vi "GEA2 Commands Dishwasher Send Receive.vi"(7 "Input Data":T2={"Source"=228, "Destination"=64, "Command"=16, "Message"=""} {"Command" format="%02x"; "Destination" format="%02x"; "Source" format="%02x"}, 11 "GEA2 Reference In 2":refnum<k24>) -> (2 "GEA2 Data":string[][](array[string]), 3 "GEA2 Reference Out 2":refnum<k24>)   [LabVIEW 2016]
uses:
  LabVIEW GEA2 Toolkit v1.0.0.0/type defs/Data In.ctl
  Type Definitions/GEA2 Commands Dishwasher.ctl
  C:/Technology Lab/NI-2010/Trunk/Utility/LabVIEW GEA2 Toolkit v1.0.0.0/Appliance.NET/GeaCommunication.dll
  LabVIEW GEA2 Toolkit v1.0.0.0/Appliance.NET/GeaCommunication.dll
  LabVIEW GEA2 Toolkit v1.0.0.0/library/GEA2_Toolkit.lvlib
panel:
  out "Dishwasher":T1
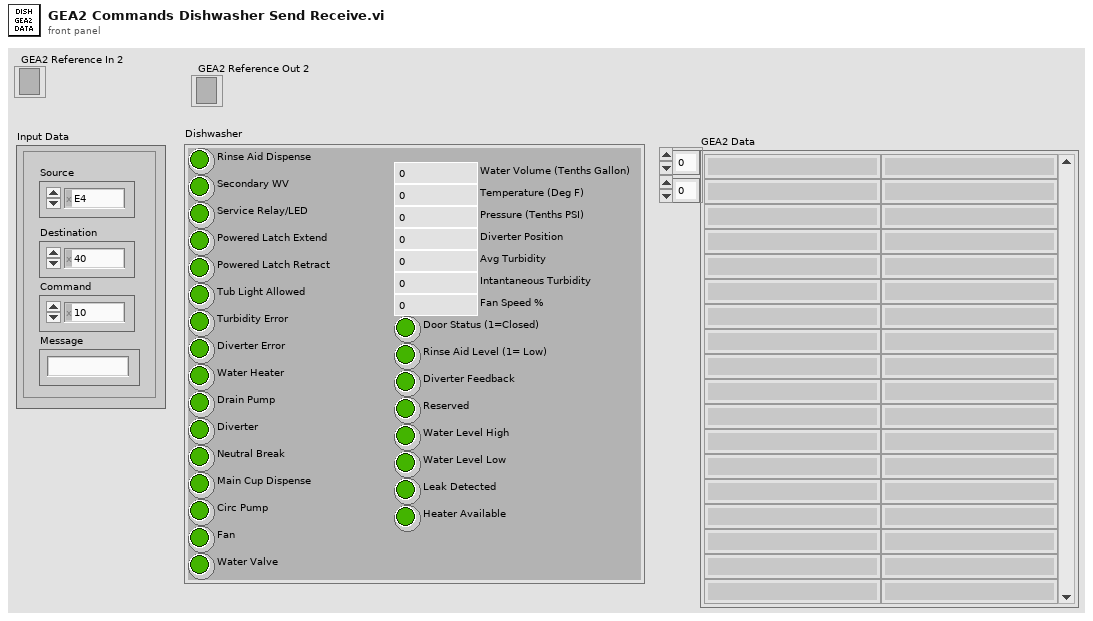
[diagram p1: front panel]
types:
  T1 = typedef "GEA2 Commands Dishwasher.ctl" = cluster{"Rinse Aid Dispense":bool, "Secondary WV":bool, "Diverter Error":bool, "Service Relay/LED":bool, "Powered Latch Extend":bool, "Powered Latch Retract":bool, "Tub Light Allowed":bool, "Turbidity Error":bool, "Water Heater":bool, "Drain Pump":bool, "Diverter":bool, "Neutral Break":bool, "Main Cup Dispense":bool, "Circ Pump":bool, "Fan":bool, "Water Valve":bool, "Water Volume (Tenths Gallon)":u8, "Temperature (Deg F)":u8, "Pressure (Tenths PSI)":u8, "Diverter Position":u8, "Avg Turbidity":u16, "Intantaneous Turbidity":u16, "Door Status (1=Closed)":bool, "Rinse Aid Level (1= Low)":bool, "Diverter Feedback":bool, "Reserved":bool, "Water Level High":bool, "Water Level Low":bool, "Leak Detected":bool, "Heater Available":bool, "Fan Speed %":u8}
  T2 = typedef "GEA2_Toolkit.lvlib/Data In.ctl" = cluster{"Source":u8, "Destination":u8, "Command":u8, "Message":string}
  T3 = typedef "GEA2_Toolkit.lvlib/Data Out.ctl" = cluster{"Source":u8, "Destination":u8, "Command":u8, "Length":u8, "CRC":u16, "Message":string}
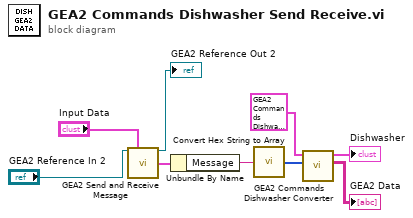
[diagram p0: block diagram]
diagram:
  n1 = call "GEA2 Send and Receive Message.vi"("GEA2 Reference In"="GEA2 Reference In 2", "Input Data"="Input Data") -> ("GEA2 Reference Out"=→"GEA2 Reference Out 2":refnum<k24>, "Converted Data Out"=w4:T3)  [unwired: 8 in, 4 out]
  n2 = Unbundle By Name(w4) -> ("Message"=w9:string)
  n3 = call "Convert Hex String to Array.vi"("Hex String In"=w9) -> ("Hex Array Out"=w8:u8[])  [unwired: 14 in]
  n4 = call "GEA2 Commands Dishwasher Converter.vi"("Data"=w8, "Dishwasher"=T1 {"Rinse Aid Dispense"=FALSE, "Secondary WV"=FALSE, "Diverter Error"=FALSE, "Service Relay/LED"=FALSE, "Powered Latch Extend"=FALSE, "Powered Latch Retract"=FALSE, "Tub Light Allowed"=FALSE, "Turbidity Error"=FALSE, "Water Heater"=FALSE, "Drain Pump"=FALSE, "Diverter"=FALSE, "Neutral Break"=FALSE, "Main Cup Dispense"=FALSE, "Circ Pump"=FALSE, "Fan"=FALSE, "Water Valve"=FALSE, "Water Volume (Tenths Gallon)"=0, "Temperature (Deg F)"=0, "Pressure (Tenths PSI)"=0, "Diverter Position"=0, "Avg Turbidity"=0, "Intantaneous Turbidity"=0, "Door Status (1=Closed)"=FALSE, "Rinse Aid Level (1= Low)"=FALSE, "Diverter Feedback"=FALSE, "Reserved"=FALSE, "Water Level High"=FALSE, "Water Level Low"=FALSE, "Leak Detected"=FALSE, "Heater Available"=FALSE, "Fan Speed %"=0}) -> ("GEA2 Data"=→"GEA2 Data":string[][], "Dishwasher Out"=→"Dishwasher":T1)  [unwired: 8 in]
